vi "nelder_make_potential_simplexes.vi"(8 "error in (no error)":errorcluster, 10 "current simplex":sgl[][](array[numeric]), 11 "parameters":T1) -> (0 "error out":errorcluster, 3 "Output Simplexes":T2)   [LabVIEW 2018]
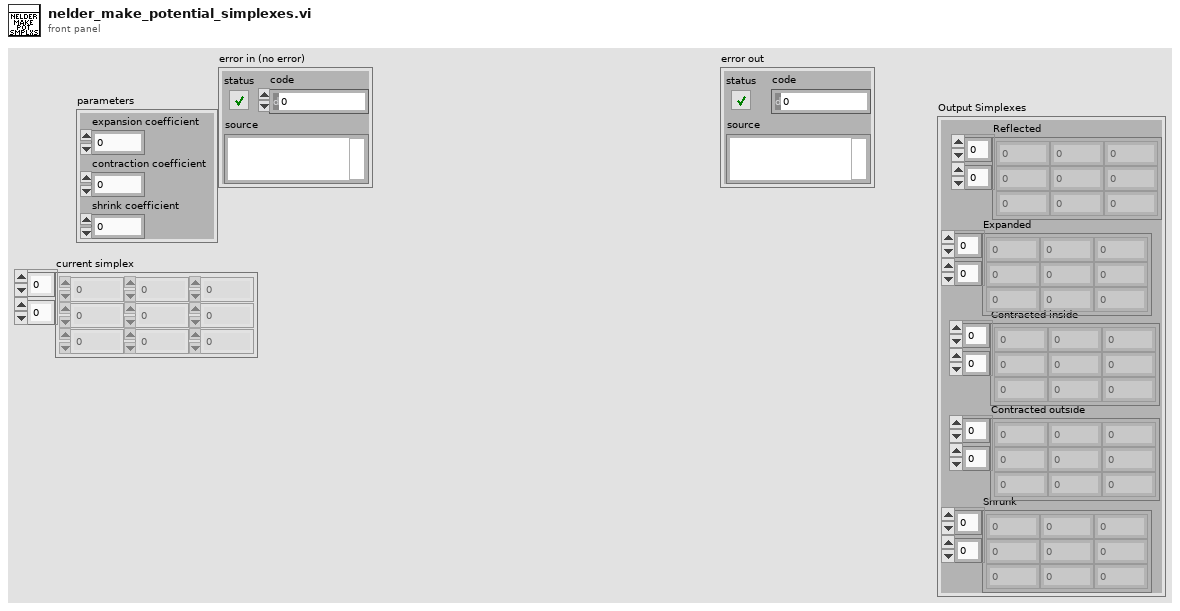
[diagram p1: front panel]
types:
  T1 = cluster{"expansion coefficient":dbl, "contraction coefficient":dbl, "shrink coefficient":dbl}
  T2 = cluster{"Reflected":sgl[][], "Expanded":sgl[][], "Contracted inside":sgl[][], "Contracted outside":sgl[][], "Shrunk":sgl[][]}
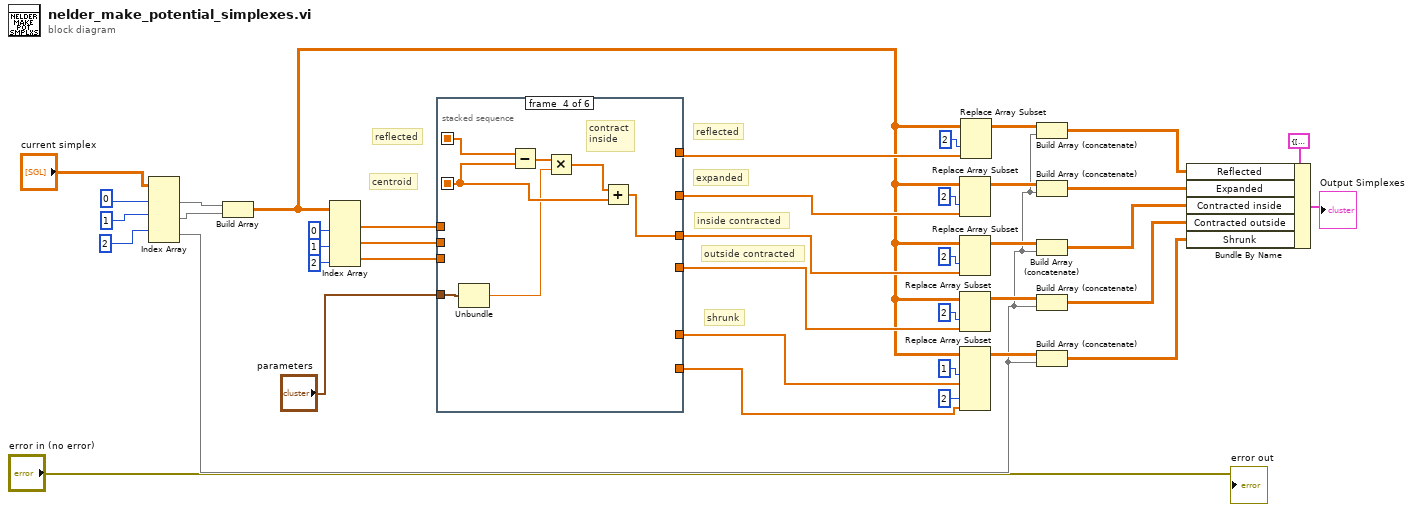
[diagram p0: block diagram]
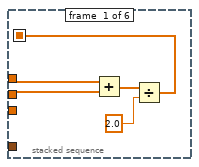
[diagram p2: hidden frame]
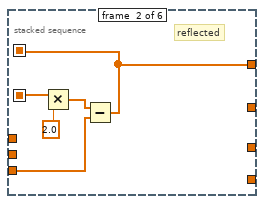
[diagram p3: hidden frame]
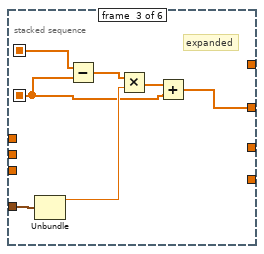
[diagram p4: hidden frame]
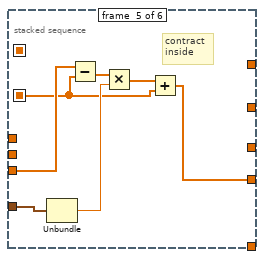
[diagram p5: hidden frame]
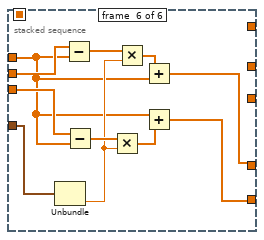
[diagram p6: hidden frame]
diagram:
  # "shrunk"
  # "outside contracted"
  # "inside contracted"
  # "expanded"
  # "reflected"
  # "centroid"
  # "reflected"
  n1 = Index Array(array="current simplex", index (row) #1=0 ("index (row)"), index (row) #2=1 ("index (row)"), index (row) #3=2) -> (element #1=w37:sgl[], element #2=w36:sgl[], element #3=w7:sgl[])  [unwired: 3 in]
  n2 = Build Array(w37, w36) -> (w18:sgl[][])
  n3 = Index Array(array=w18, index (col) #1=0 ("disabled index (col)"), index (col) #2=1 ("index (col)"), index (col) #3=2 ("index (col)")) -> (element #1=w30:sgl[], element #2=w29:sgl[], element #3=w28:sgl[])  [unwired: 3 in]
  n4 = stacked-sequence {
    seq-local: [w41 _ _ _ _ _] -> [_ w50 w52 w60 w66 _]
    seq-local: [_ w46 _ _ _ _] -> [_ _ w56 w64 _ _]
    tunnel: w30 -> [w44 _ _ _ _ w74]
    tunnel: w29 -> [w45 _ _ _ _ w82]
    tunnel: w28 -> [_ w47 _ _ w71 w81]
    tunnel: "parameters" -> [_ _ w57 w62 w69 w78]
    tunnel: [_ w46 _ _ _ _] -> w22
    tunnel: [_ _ w51 _ _ _] -> w21
    tunnel: [_ _ _ w59 _ _] -> w20
    tunnel: [_ _ _ _ w65 _] -> w19
    tunnel: [_ _ _ _ _ w73] -> w14
    tunnel: [_ _ _ _ _ w72] -> w15
    frame #0 {
      n5 = Add(x=w44, y=w45) -> (x+y=w43:sgl[])
      n6 = Divide(x=w43, y=2.0) -> (x/y=w41:dbl[])
    }
    frame #1 {
      # "reflected"
      n7 = Multiply(x=w50, y=2.0) -> (x*y=w48:dbl[])
      n8 = Subtract(x=w48, y=w47) -> (x-y=w46:dbl[])
    }
    frame #2 {
      # "expanded"
      n9 = Unbundle(w57) -> ("expansion coefficient"=w54:dbl)  [unwired: 2 out]
      n10 = Subtract(x=w56, y=w52) -> (x-y=w55:dbl[])
      n11 = Multiply(x=w55, y=w54) -> (x*y=w53:dbl[])
      n12 = Add(x=w53, y=w52) -> (x+y=w51:dbl[])
    }
    frame #3 {
      # "contract\ninside"
      n13 = Unbundle(w62) -> ("contraction coefficient"=w58:dbl)  [unwired: 2 out]
      n14 = Subtract(x=w64, y=w60) -> (x-y=w63:dbl[])
      n15 = Multiply(x=w63, y=w58) -> (x*y=w61:dbl[])
      n16 = Add(x=w61, y=w60) -> (x+y=w59:dbl[])
    }
    frame #4 {
      # "contract \ninside"
      n17 = Unbundle(w69) -> ("contraction coefficient"=w68:dbl)  [unwired: 2 out]
      n18 = Subtract(x=w71, y=w66) -> (x-y=w70:dbl[])
      n19 = Multiply(x=w70, y=w68) -> (x*y=w67:dbl[])
      n20 = Add(x=w67, y=w66) -> (x+y=w65:dbl[])
    }
    frame #5 {
      n21 = Unbundle(w78) -> ("shrink coefficient"=w77:dbl)  [unwired: 2 out]
      n22 = Subtract(x=w82, y=w74) -> (x-y=w79:sgl[])
      n23 = Subtract(x=w81, y=w74) -> (x-y=w80:sgl[])
      n24 = Multiply(x=w80, y=w77) -> (x*y=w75:dbl[])
      n25 = Multiply(x=w79, y=w77) -> (x*y=w76:dbl[])
      n26 = Add(x=w76, y=w74) -> (x+y=w72:dbl[])
      n27 = Add(x=w74, y=w75) -> (x+y=w73:dbl[])
    }
  }
  n28 = Replace Array Subset(array=w18, new element=w21, index (col)=2 ("disabled index (col)")) -> (w11:sgl[][])  [unwired: 1 in]
  n29 = Replace Array Subset(array=w18, new element=w20, index (col)=2 ("disabled index (col)")) -> (w10:sgl[][])  [unwired: 1 in]
  n30 = Replace Array Subset(array=w18, new element=w19, index (col)=2 ("disabled index (col)")) -> (w9:sgl[][])  [unwired: 1 in]
  n31 = Replace Array Subset(array=w18, new element #1=w15, index (col) #1=1 ("disabled index (col)"), new element #2=w14, index (col) #2=2 ("index (col)")) -> (w8:sgl[][])  [unwired: 2 in]
  n32 = Replace Array Subset(array=w18, new element=w22, index (col)=2 ("disabled index (col)")) -> (w12:sgl[][])  [unwired: 1 in]
  n33 = Build Array (concatenate)(w12, w7) -> (w2:sgl[][])
  n34 = Build Array (concatenate)(w11, w7) -> (w3:sgl[][])
  n35 = Build Array (concatenate)(w10, w7) -> (w4:sgl[][])
  n36 = Build Array (concatenate)(w9, w7) -> (w5:sgl[][])
  n37 = Build Array (concatenate)(w8, w7) -> (w6:sgl[][])
  n38 = Bundle By Name(cluster=T2 {"Reflected"=[], "Expanded"=[], "Contracted inside"=[], "Contracted outside"=[], "Shrunk"=[]} ("output"), "Reflected"=w2, "Expanded"=w3, "Contracted inside"=w4, "Contracted outside"=w5, "Shrunk"=w6) -> (→"Output Simplexes":T2)
  "error out" <- "error in (no error)"
